vi "CRYRun Project.vi"(2 "Calibrate? (F)":bool, 12 "Do not display panel (F)":bool) -> ()   [LabVIEW 2013]
uses:
  Typedef Control/CRYResult Cluster.ctl
  Typedef Control/CRYTS.ctl
  Typedef Control/CRYStep.ctl
  CRYProject Run Control Global.vi
  Data/CRYData & result stacks global.vi
  CRYMainGlobal.vi
  Calibration/SubVI/CRYCal Global.vi
  CRYProject/CRYProject Editor Global.vi
  Misc/SubVI/CRYMisc vis settings global.vi
  CRYWindow/SubVI/CRYMain Sub Window Global.vi
  Statistics/CRYStatistics Global.vi
panel:
  out "Seq running Ref":refnum<vi>
  out "Seq cont border Ref":refnum<vi>
  out "Seq Continue Ref":refnum<vi>
  out "Verdict Ref":refnum<vi>
  out "Margin Ref":refnum<vi>
  out "Category Name Ref":refnum<vi>
  in  "Updateflg":bool
  in  "VerdictLabel":string
  out "Elapsed Ref":refnum<vi>
  in  "Time Out":bool
  out "Step Name":string
  in  "Verdict":bool caption="°¬ü¬,1Áõ¬,äÂ(Ó"
  out "Step Setup VI No":u32
  out "Margin":dbl format="%#_6p"
  out "Category Name":string
  out "Project Name":string
  in  "done call":bool
  in  "Abort":bool
  in  "Continue":bool
  in  "running":bool
  out "cont border":bool
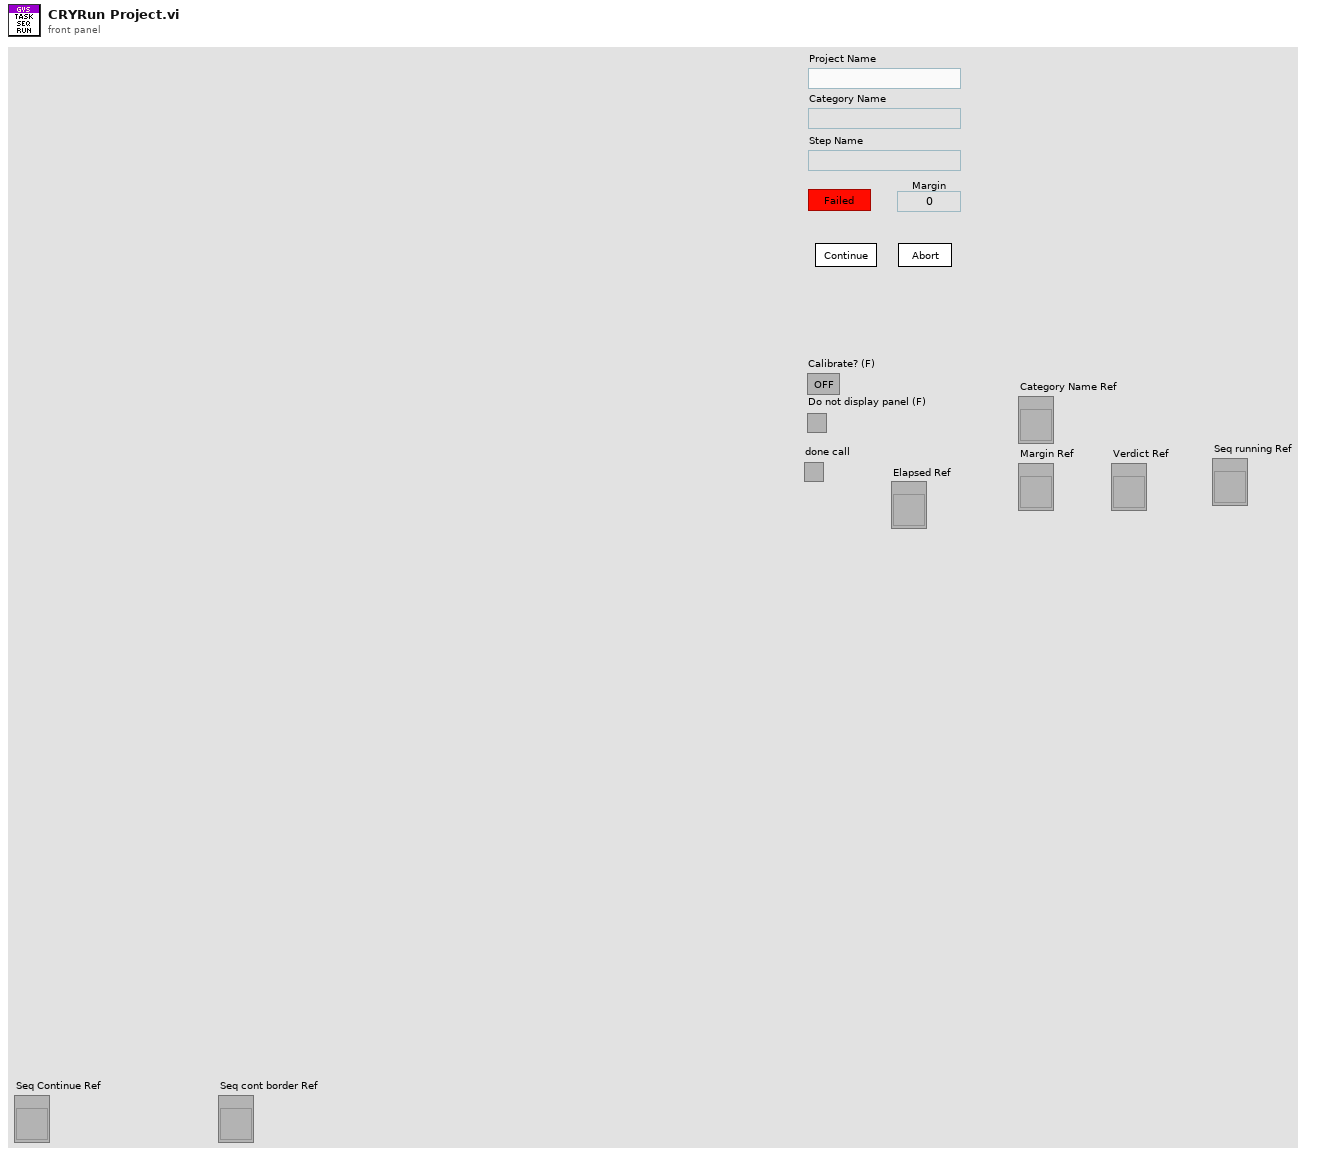
[diagram p1: front panel]
types:
  T1 = typedef "CRYStep.ctl" = cluster{"No.VI":i32, "Category":string, "StepName":string, "Seq setup flattened":string, "Comment":string, "Steps config.":bool[], "Jump config":i32[], "Start":dbl, "Increment":dbl, "Name":string, "Unit":string, "Y data":u16, "Y prefix":string, "Y dB ref":dbl, "Y unit":string, "Repeat State Array":cluster{"Start":dbl, "Increment":dbl, "Count":i32, "Num":i32}[]}
  T2 = typedef "CRYTS.ctl" = cluster{"No.TS":u16, "TS File Path":path, "TS Name":string, "EditStepName":string, "Steps":T1[], "New State":bool, "Change State":bool, "Flattened CurveLib Data":string, "Document Data":string, "EditStepNo":u16, "Operator Start File":string, "Sequence Type":string, "Sequence Language":string}
  T3 = cluster{"Category Name Ref":refnum<vi>, "Step Name Ref":refnum<vi>, "Verdict Ref":refnum<vi>, "Seq Continue Ref":refnum<vi>, "Seq cont border Ref":refnum<vi>, "Seq running Ref":refnum<vi>}
  T4 = typedef "CRYStart Cluster.ctl" = cluster{"SequenceName":string, "Preload Stimulus":bool, "CloseOpenedDisplay":bool, "ClearMeasuredData":bool, "UpdateDisplayDuringRun":bool, "DisplayForConfirmation":bool, "HaltOnFail":bool, "UseSameHardware":bool, "UseSameCalibration":bool}
  T5 = typedef "CRYResult Cluster.ctl" = cluster{"Name":string, "Margin":dbl, "unit":string, "Verdict":bool, "Limit":string, "Max/Min":string, "protected":bool, "Step No.":i32, "Test Info":string, "AutoProtect":bool}
  T6 = typedef "GVSResult Cluster.ctl" = cluster{"Name":string, "Margin":dbl, "unit":string, "Verdict":bool, "Limit":string, "Max/Min":string, "protected":bool, "Step No.":i32, "Test Info":string, "AutoProtect":bool}
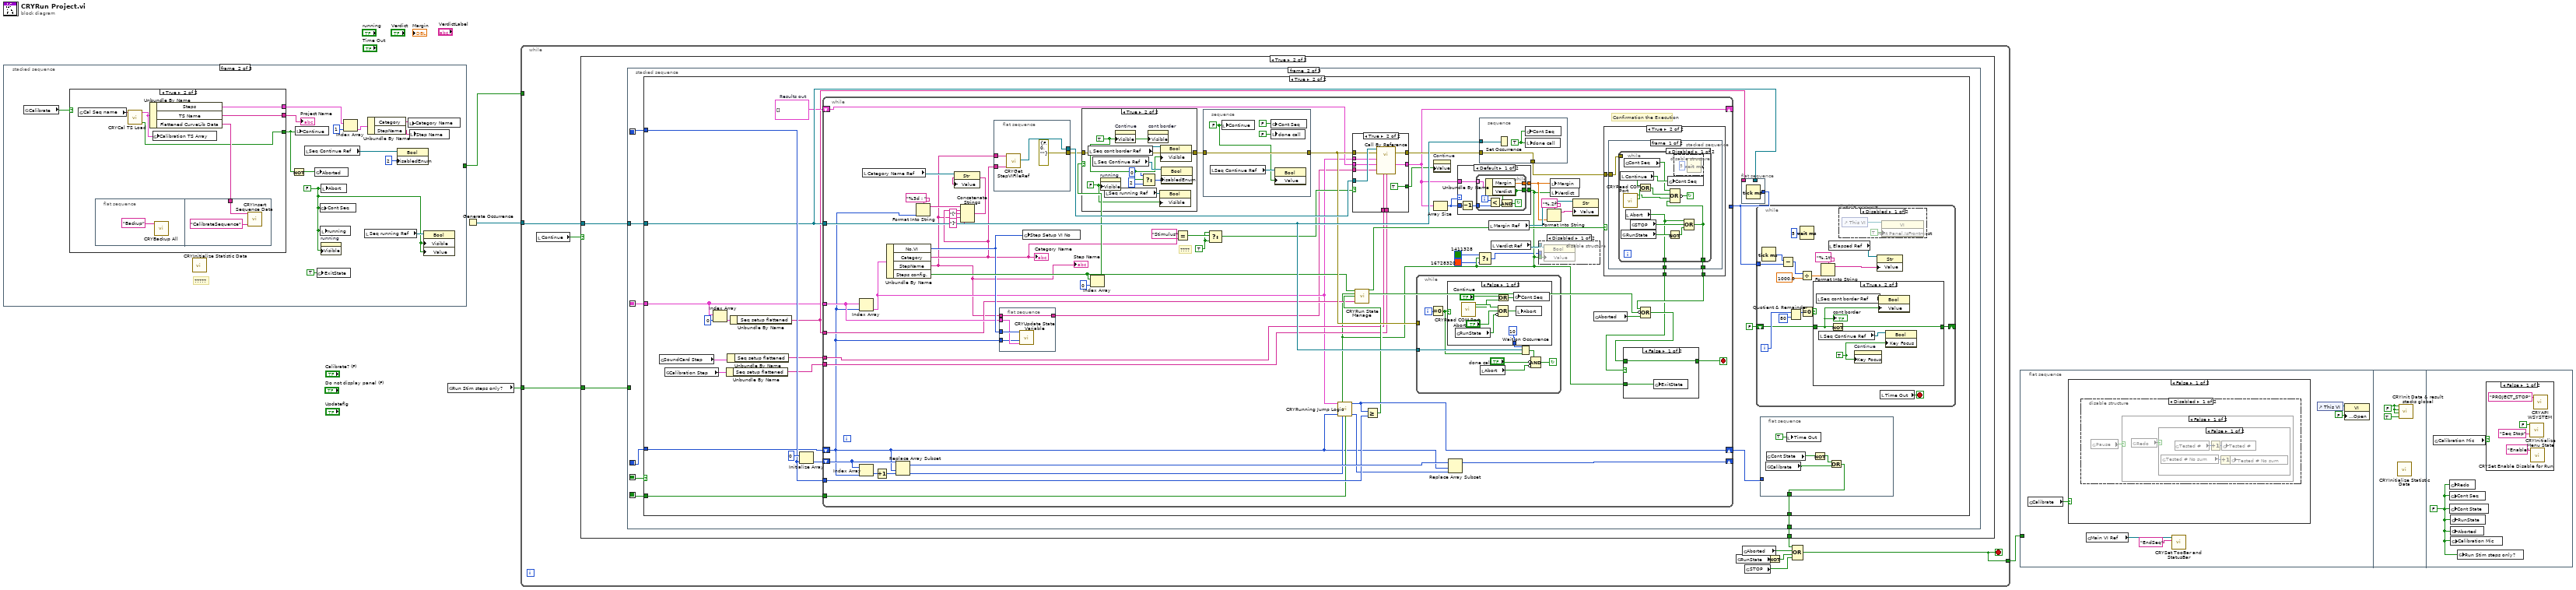
[diagram p0: block diagram]
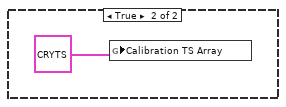
[diagram p5: hidden frame]
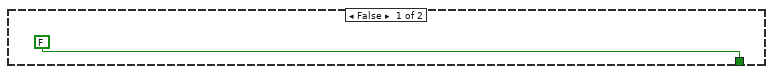
[diagram p7: hidden frame]
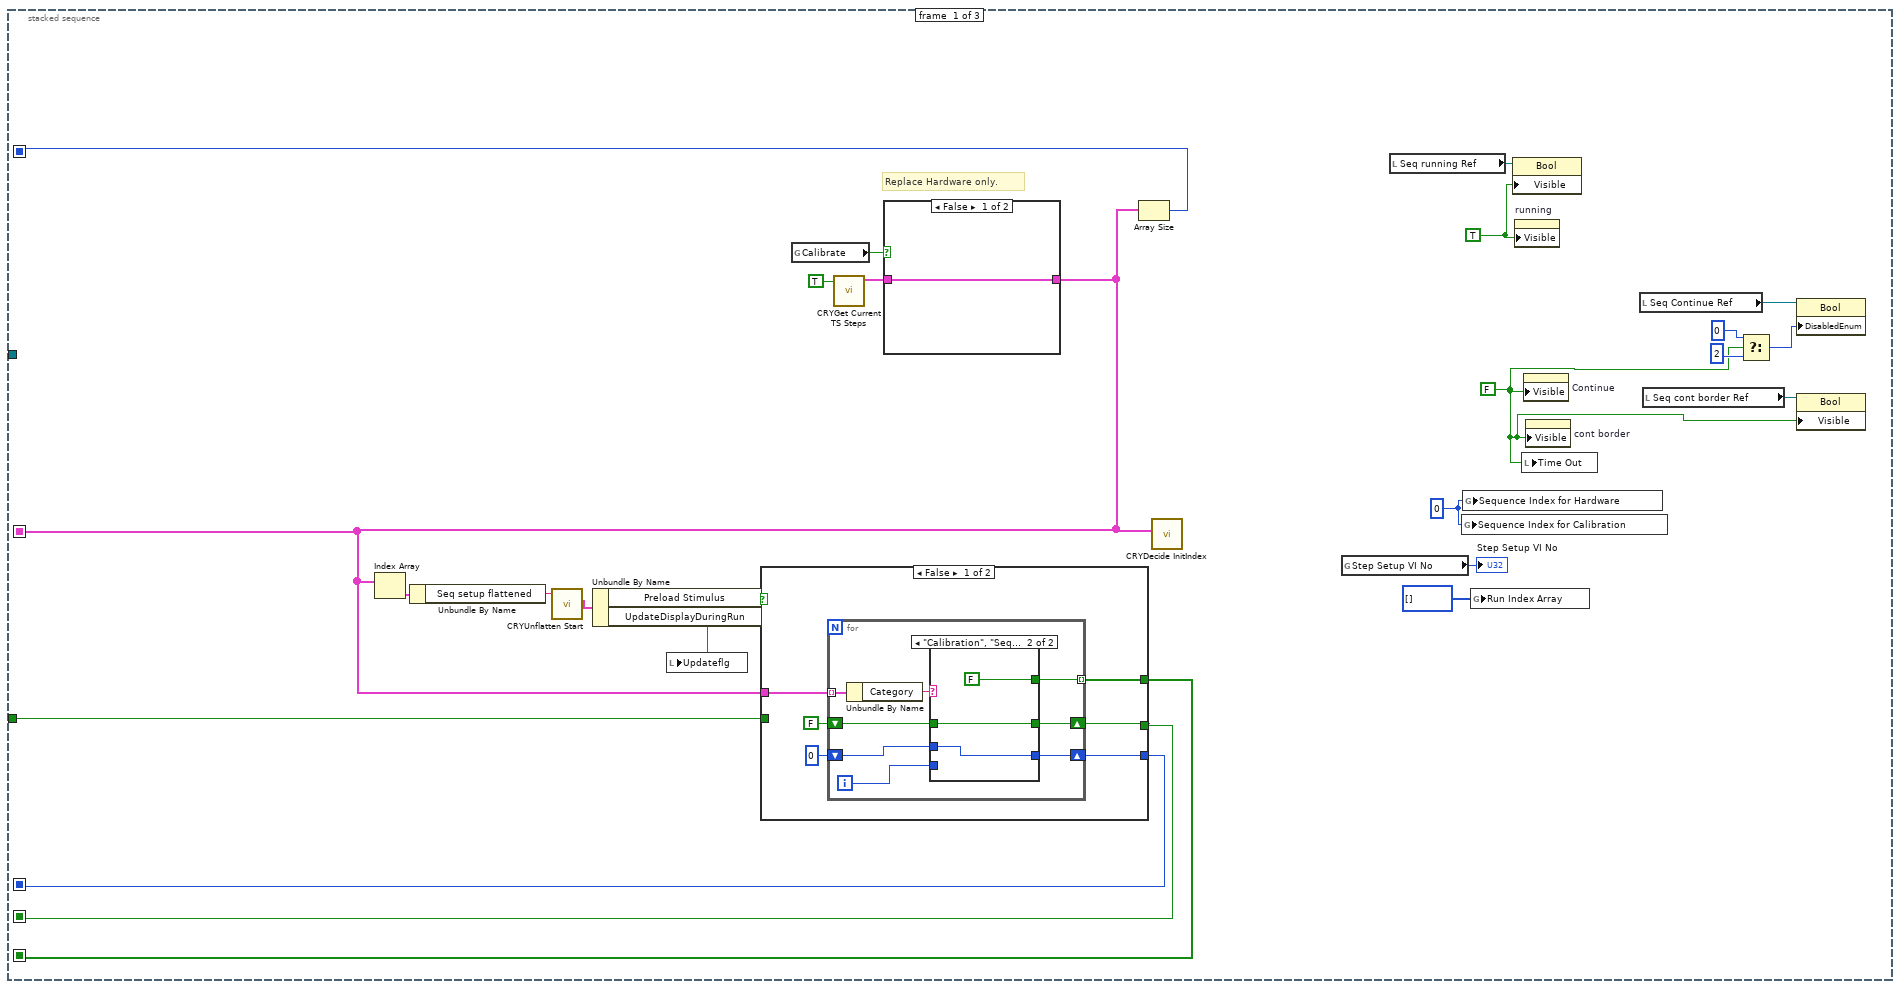
[diagram p8: hidden frame]
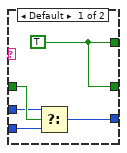
[diagram p9: hidden frame]
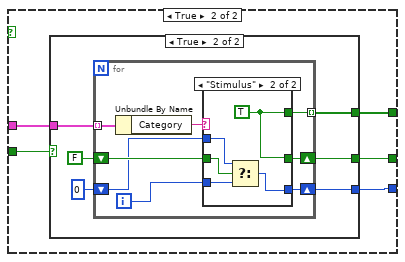
[diagram p10: hidden frame]
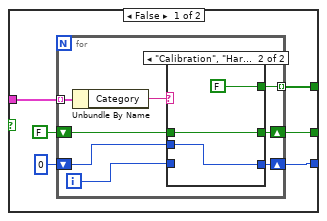
[diagram p11: hidden frame]
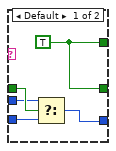
[diagram p12: hidden frame]
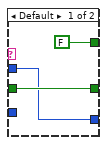
[diagram p13: hidden frame]
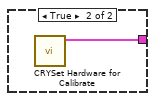
[diagram p14: hidden frame]
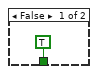
[diagram p15: hidden frame]
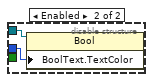
[diagram p18: hidden frame]
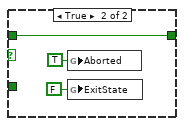
[diagram p19: hidden frame]
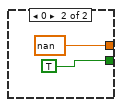
[diagram p20: hidden frame]
diagram:
  n1 = stacked-sequence {
    tunnel: [_ _ w71] -> w3
    frame #0 {
      w11 = TRUE ("Verdict")
      n2 = control-ref of="This VI"() -> (w10:refnum<vi>)
      n3 = call "CRYSet Run Project Front Panel.vi"("Vi Ref in"=w10) -> ()  [unwired: 10 in, 1 out]
      n4 = call "CRYOperator Process.vi"("sAction"="RunCloseAll") -> ()  [unwired: 10 in, 1 out]
      n5 = local write "Verdict"(w11) -> ()
      n6 = global write "CRYProject Run Control Global.vi" "RunState"(w11) -> ()
      n7 = global read "CRYCal Global.vi" "Calibration Mic"() -> (w7:bool)
      n8 = control-ref of="Abort"() -> (w9:refnum<vi>)
      n9 = control-ref of="Continue"() -> (w8:refnum<vi>)
      n10 = global write "CRYData & result stacks global.vi" "Tested # No sum"(u16 0 ("Tested # No sum")) -> ()
      n11 = global write "CRYMainGlobal.vi" "Seq Continue Ref"(w8) -> ()
      n12 = global write "CRYMainGlobal.vi" "Seq Abort Ref"(w9) -> ()
      n13 = case shown="False" w7 {
        frame False {
          n14 = call "CRYInitialize Menu State.vi"("sAction"="Seq Run", "Is Disable?"=TRUE) -> ()  [unwired: 10 in]
          n15 = call "CRYAPI WSYSTEM.vi"("sAction"="PROJECT_RUN") -> ()  [unwired: 7 in, 4 out]
          n16 = call "CRYSet Enable Disable for Run.vi"("sOption"="Disable") -> ()  [unwired: 15 in]
        }
        frame True {
        }
      }
    }
    frame #1 {
      w19 = FALSE
      # "?????"
      n17 = global read "CRYCal Global.vi" "Calibrate"() -> (w29:bool)
      n18 = case shown="True" w29 {
        tunnel: [TRUE ("cont button") w50] -> w17
        tunnel: [w32 w54] -> w27
        tunnel: [w33 w53] -> w28
        frame False {
          n19 = call "CRYGet Current TS Steps.vi"() -> ("TS Name"=w33:string, "Steps"=w32:T1[])  [unwired: 7 in, 3 out]
          n20 = for {
            tunnel: w32 -> [w36] mode=indexing
            shift-right: [w41] -> w30
            shift-left: i32[] [] -> [w40]
            n21 = Unbundle By Name(w36) -> ("Category"=w43:string, "No.VI"=w42:i32, "Steps config."=w39:bool[], "Start"=w35:dbl)
            n22 = Index Array(array=w39, index=6) -> (element=w37:bool)
            n23 = case shown="Default" w43 {
              tunnel: w42 -> [w47 _]
              tunnel: [w46 w49] -> w41
              tunnel: w40 -> [w48 w49]
              frame Default {
                n24 = Build Array (concatenate)(w48, w47) -> (w46:i32[])
              }
              frame "Calibration", "Stimulus" {
              }
            }
            n25 = case shown="True" w37 {
              tunnel: w36 -> [_ w45]
              tunnel: w35 -> [_ w44]
              frame False {
              }
              frame True {
                n26 = call "CRYUpdate Curve from Jump.vi"("Y Value"=w44, "Step Configure"=w45) -> ()  [unwired: 9 in, 1 out]
              }
            }
          }
          n27 = call "CRYDelete Step Data.vi"("Step No"=w30) -> ()  [unwired: 11 in]
        }
        frame True {
          n28 = global read "CRYCal Global.vi" "Cal Seq name"() -> (w55:string)
          n29 = flat-sequence {
            tunnel: w51 -> [w58]
            frame #0 {
              n30 = call "CRYBackup All.vi"("sOption"="Backup") -> ()  [unwired: 11 in]
            }
            frame #1 {
              n31 = call "CRYInsert Sequence Data.vi"("sOption"="CalibrateSequence", "sFlattenedCurveData"=w58) -> ()  [unwired: 8 in, 2 out]
            }
          }
          n32 = call "CRYCal TS Load.vi"("Cal seq name"=w55) -> ("Cal sequence"=w52:T2, "status"=w50:bool)  [unwired: 8 out]
          n33 = Unbundle By Name(w52) -> ("Steps"=w54:T1[], "TS Name"=w53:string, "Flattened CurveLib Data"=w51:string)
          n34 = global write "CRYProject Editor Global.vi" "Calibration TS Array"(w52) -> ()
        }
      }
      "Project Name" <- w28
      n35 = call "CRYInitialize Statistic Data.vi"() -> ()  [unwired: 12 in]
      n36 = Not(x=w17) -> (.not. x?=w16:bool)
      n37 = local write "Continue"(w17) -> ()
      n38 = local read "Seq Continue Ref"() -> (w21:refnum<vi>)
      n39 = global write "CRYProject Run Control Global.vi" "Aborted"(w16) -> ()
      n40 = global write "CRYProject Run Control Global.vi" "ExitState"(TRUE ("ExitState")) -> ()
      n41 = global write "CRYProject Run Control Global.vi" "Cont Seq"(w19) -> ()
      n42 = local write "running"(w19) -> ()
      n43 = property on="running" class="Bool (strict)"("Visible"=w19) -> ()  [unwired: 2 in, 2 out]
      n44 = local write "Abort"(w19) -> ()
      n45 = Index Array(array=w27, index=1) -> (element=w24:T1)
      n46 = local read "Seq running Ref"() -> (w20:refnum<vi>)
      n47 = Unbundle By Name(w24) -> ("Category"=w23:string, "StepName"=w22:string)
      n48 = property class="Bool"(reference=w21, "DisabledEnum"=u8 2) -> ()  [unwired: 1 in, 2 out]
      n49 = local write "Category Name"(w23) -> ()
      n50 = local write "Step Name"(w22) -> ()
      n51 = property class="Bool"(reference=w20, "Visible"=w19, "Value"=w19) -> ()  [unwired: 1 in, 2 out]
    }
    frame #2 {
      n52 = global read "CRYCal Global.vi" "Calibrate"() -> (w71:bool)
      n53 = global write "CRYMisc vis settings global.vi" "Menu?"(FALSE ("Menu?")) -> ()
      n54 = global read "CRYMain Sub Window Global.vi" "Main VI Ref"() -> (w70:refnum<vi>)
      n55 = call "CRYSet TooBar and StatusBar.vi"("Type"="StartSeq", "MainVI Ref In"=w70) -> ("output cluster"=w67:T3, "Elapsed Ref"=→"Elapsed Ref":refnum<vi>)  [unwired: 7 in, 1 out]
      n56 = local read "Verdict"() -> (w64:bool)
      n57 = Unbundle(w67) -> ("Category Name Ref"=→"Category Name Ref":refnum<vi>, "Step Name Ref"=→"Margin Ref":refnum<vi>, "Verdict Ref"=w63:refnum<vi>, "Seq Continue Ref"=→"Seq Continue Ref":refnum<vi>, "Seq cont border Ref"=→"Seq cont border Ref":refnum<vi>, "Seq running Ref"=→"Seq running Ref":refnum<vi>)
      "Verdict Ref" <- w63
      n58 = property class="Bool"(reference=w63, "Value"=w64) -> ()  [unwired: 1 in, 2 out]
      n59 = property on="Verdict" class="Bool (strict)"() -> ("Strings [4]"=w62:string[])  [unwired: 2 in, 2 out]
      n60 = property class="Bool"(reference=w63, "Strings [4]"=w62) -> ()  [unwired: 1 in, 2 out]
    }
  }
  n61 = global read "CRYProject Run Control Global.vi" "Run Stim steps only?"() -> (w2:bool)
  n62 = Generate Occurrence() -> (w4:refnum<k4>)
  n63 = while {
    tunnel: w4 -> [w81]
    tunnel: w3 -> [_]
    tunnel: w2 -> [w74]
    tunnel: [w73] -> w1
    stop <- w73 stop-if-true
    n64 = local read "Continue"() -> (w80:bool)
    n65 = case shown="True" w80 {
      tunnel: w81 -> [_ w85]
      tunnel: [FALSE ("abort button") w84] -> w76
      tunnel: w74 -> [_ w83]
      frame False {
      }
      frame True {
        n66 = stacked-sequence {
          seq-local: [w106 _ _] -> [_ w187 _]
          seq-local: [w86 _ _] -> [_ w189 _]
          seq-local: [w100 _ _] -> [_ w186 _]
          seq-local: [w98 _ _] -> [_ w185 _]
          seq-local: [w96 _ _] -> [_ w184 _]
          tunnel: w85 -> [_ w190 _]
          tunnel: [_ w188 _] -> w84
          tunnel: w83 -> [w99 _ _]
          frame #0 {
            w105 = 0 ("Sequence Index for Hardware")
            w88 = FALSE ("Visible")
            w91 = TRUE ("Visible")
            # "Replace Hardware only."
            n67 = global read "CRYCal Global.vi" "Calibrate"() -> (w109:bool)
            n68 = call "CRYGet Current TS Steps.vi"("Current Only?"=TRUE) -> ("Steps"=w108:T1[])  [unwired: 6 in, 4 out]
            n69 = case shown="False" w109 {
              tunnel: [w182 w183] -> w86
              tunnel: w108 -> [w182 _]
              frame False {
              }
              frame True {
                n70 = call "CRYSet Hardware for Calibrate.vi"() -> ("Steps Out"=w183:T1[])  [unwired: 11 in]
              }
            }
            n71 = Index Array(array=w86) -> (element=w104:T1)  [unwired: 1 in]
            n72 = Unbundle By Name(w104) -> ("Seq setup flattened"=w103:string)
            n73 = call "CRYUnflatten Start.vi"("Unflatten Sequence"=w103) -> ("Sequence Configure"=w102:T4)  [unwired: 8 in, 2 out]
            n74 = Unbundle By Name(w102) -> ("Preload Stimulus"=w101:bool, "UpdateDisplayDuringRun"=w97:bool)
            n75 = local write "Updateflg"(w97) -> ()
            n76 = case shown="False" w101 {
              tunnel: w86 -> [w116 w136]
              tunnel: [w115 w135] -> w100
              tunnel: w99 -> [_ w137]
              tunnel: [w113 w134] -> w98
              tunnel: [w111 w133] -> w96
              frame False {
                n77 = for {
                  tunnel: w116 -> [w124] mode=indexing
                  tunnel: [w122] -> w115 mode=indexing
                  shift-right: [w120] -> w113
                  shift-left: FALSE -> [w121]
                  shift-right: [w118] -> w111
                  shift-left: 0 -> [w117]
                  i -> [w119]
                  n78 = Unbundle By Name(w124) -> ("Category"=w123:string)
                  n79 = case shown="\"Calibration\", \"Sequence\", \"SoundCard\"" w123 {
                    tunnel: [w129 FALSE] -> w122
                    tunnel: w121 -> [w128 w131]
                    tunnel: [w129 w131] -> w120
                    tunnel: w119 -> [w127 _]
                    tunnel: [w126 w130] -> w118
                    tunnel: w117 -> [w125 w130]
                    frame Default {
                      w129 = TRUE
                      n80 = Select(t=w125, s=w128, f=w127) -> (s? t:f=w126:i32)
                    }
                    frame "Calibration", "Sequence", "SoundCard" {
                    }
                  }
                }
              }
              frame True {
                n81 = case shown="True" w137 {
                  tunnel: w136 -> [w143 w165]
                  tunnel: [w142 w164] -> w135
                  tunnel: [w140 w162] -> w134
                  tunnel: [w138 w160] -> w133
                  frame False {
                    n82 = for {
                      tunnel: w143 -> [w151] mode=indexing
                      tunnel: [w149] -> w142 mode=indexing
                      shift-right: [w147] -> w140
                      shift-left: FALSE -> [w148]
                      shift-right: [w144] -> w138
                      shift-left: 0 -> [w145]
                      i -> [w146]
                      n83 = Unbundle By Name(w151) -> ("Category"=w150:string)
                      n84 = case shown="\"Calibration\", \"Hardware\", \"Sequence\", \"Stimulus\"" w150 {
                        tunnel: [w156 FALSE] -> w149
                        tunnel: w148 -> [w155 w158]
                        tunnel: [w156 w158] -> w147
                        tunnel: w146 -> [w154 _]
                        tunnel: w145 -> [w153 w157]
                        tunnel: [w152 w157] -> w144
                        frame Default {
                          w156 = TRUE
                          n85 = Select(t=w153, s=w155, f=w154) -> (s? t:f=w152:i32)
                        }
                        frame "Calibration", "Hardware", "Sequence", "Stimulus" {
                        }
                      }
                    }
                  }
                  frame True {
                    n86 = for {
                      tunnel: w165 -> [w173] mode=indexing
                      tunnel: [w171] -> w164 mode=indexing
                      shift-right: [w169] -> w162
                      shift-left: FALSE -> [w170]
                      shift-right: [w166] -> w160
                      shift-left: 0 -> [w167]
                      i -> [w168]
                      n87 = Unbundle By Name(w173) -> ("Category"=w172:string)
                      n88 = case shown="\"Stimulus\"" w172 {
                        tunnel: [FALSE w181] -> w171
                        tunnel: w170 -> [w175 w180]
                        tunnel: [w175 w181] -> w169
                        tunnel: w168 -> [_ w179]
                        tunnel: w167 -> [w174 w178]
                        tunnel: [w174 w177] -> w166
                        frame Default {
                        }
                        frame "Stimulus" {
                          w181 = TRUE
                          n89 = Select(t=w178, s=w180, f=w179) -> (s? t:f=w177:i32)
                        }
                      }
                    }
                  }
                }
              }
            }
            n90 = Array Size(array=w86) -> (size(s)=w106:i32)
            n91 = call "CRYDecide InitIndex.vi"("Steps In"=w86) -> ()  [unwired: 11 in]
            n92 = global read "CRYProject Editor Global.vi" "Step Setup VI No"() -> (→"Step Setup VI No":i32)
            n93 = local read "Seq running Ref"() -> (w92:refnum<vi>)
            n94 = global write "CRYProject Editor Global.vi" "Sequence Index for Calibration"(w105) -> ()
            n95 = global write "CRYProject Editor Global.vi" "Sequence Index for Hardware"(w105) -> ()
            n96 = global write "CRYProject Run Control Global.vi" "Run Index Array"(u32[] [] ("Run Index Array")) -> ()
            n97 = property class="Bool"(reference=w92, "Visible"=w91) -> ()  [unwired: 1 in, 2 out]
            n98 = property on="running" class="Bool (strict)"("Visible"=w91) -> ()  [unwired: 2 in, 2 out]
            n99 = local write "Time Out"(w88) -> ()
            n100 = property on="Continue" class="Bool (strict)"("Visible"=w88) -> ()  [unwired: 2 in, 2 out]
            n101 = property on="cont border" class="Bool (strict)"("Visible"=w88) -> ()  [unwired: 2 in, 2 out]
            n102 = local read "Seq Continue Ref"() -> (w94:refnum<vi>)
            n103 = local read "Seq cont border Ref"() -> (w93:refnum<vi>)
            n104 = Select(t=u8 0, s=w88, f=u8 2) -> (s? t:f=w87:u8)
            n105 = property class="Bool"(reference=w94, "DisabledEnum"=w87) -> ()  [unwired: 1 in, 2 out]
            n106 = property class="Bool"(reference=w93, "Visible"=w88) -> ()  [unwired: 1 in, 2 out]
          }
          frame #1 {
            n107 = case shown="True" w185 {
              tunnel: w190 -> [_ w203]
              tunnel: w189 -> [_ w198]
              tunnel: [TRUE w210] -> w188
              tunnel: w187 -> [_ w207]
              tunnel: w186 -> [_ w206]
              tunnel: w184 -> [_ w205]
              frame False {
              }
              frame True {
                w200 = T5[] []  # Results out
                n108 = global read "CRYProject Editor Global.vi" "SoundCard Step"() -> (w194:T1)
                n109 = global read "CRYProject Editor Global.vi" "Calibration Step"() -> (w195:T1)
                n110 = Index Array(array=w198, index=0) -> (element=w201:T1)
                n111 = Unbundle By Name(w195) -> ("Seq setup flattened"=w192:string)
                n112 = Unbundle By Name(w194) -> ("Seq setup flattened"=w193:string)
                n113 = Unbundle By Name(w201) -> ("Seq setup flattened"=w199:string)
                n114 = Initialize Array(0 ("step execution\ncounter"), w207) -> (w208:i32[])
                n115 = while {
                  tunnel: w203 -> [w295]
                  tunnel: w198 -> [w273]
                  shift-right: [w283] -> w204
                  shift-left: w205 -> [w237]
                  tunnel: w207 -> [w282]
                  shift-right: [w271] -> _
                  shift-left: w208 -> [w286]
                  tunnel: w206 -> [w281]
                  tunnel: w199 -> [w261]
                  shift-right: [w260] -> _
                  shift-left: w200 -> [w259]
                  tunnel: w193 -> [w258]
                  tunnel: w192 -> [w257]
                  tunnel: w197 -> [_]
                  stop <- w267 stop-if-true
                  w262 = TRUE
                  # "????"
                  # "Confirmation the Execution"
                  n116 = Index Array(array=w273, index=w237) -> (element=w256:T1)
                  n117 = Index Array(array=w286, index=w237) -> (element=w287:i32)
                  n118 = local read "Category Name Ref"() -> (w254:refnum<vi>)
                  n119 = Increment(x=w287) -> (x+1=w284:i32)
                  n120 = Unbundle By Name(w256) -> ("No.VI"=w274:i32, "Category"=w251:string, "StepName"=w236:string, "Steps config."=w279:bool[])
                  "Category Name" <- w251
                  "Step Name" <- w236
                  n121 = Replace Array Subset(array=w286, new element=w284, index=w237) -> (w285:i32[])
                  n122 = Format Into String(format string="%3d : ", w237) -> (resulting string=w240:string)  [unwired: 2 in, 1 out]
                  n123 = Concatenate Strings(w240, w251, "[" ("string"), w236, "]" ("string")) -> (w248:string)
                  n124 = property class="Str"(reference=w254, "Value"=w248) -> ()  [unwired: 1 in, 2 out]
                  n125 = flat-sequence {
                    tunnel: [w312] -> w294
                    tunnel: [errorcluster {"status"=FALSE, "code"=0, "source"=""} ("error out")] -> w291
                    tunnel: w251 -> [w310]
                    tunnel: w236 -> [w309]
                    frame #0 {
                      n126 = call "CRYGet StepVIFileRef.vi"("Category"=w310, "Step Name"=w309) -> ("Step Run VI ref"=w312:refnum<vi>)  [unwired: 6 in, 2 out]
                    }
                  }
                  n127 = flat-sequence {
                    tunnel: w274 -> [w308]
                    tunnel: w273 -> [w307]
                    tunnel: w237 -> [w306]
                    tunnel: w236 -> [w305]
                    tunnel: [w305] -> w255
                    frame #0 {
                      n128 = call "CRYUpdate State Variable.vi"("Step VI No In"=w308, "Step Index"=w306, "Steps"=w307) -> ()  [unwired: 12 in, 1 out]
                    }
                  }
                  n129 = global write "CRYProject Editor Global.vi" "Step Setup VI No"(w274) -> ()
                  n130 = Index Array(array=w279, index=0) -> (element=w278:bool)
                  n131 = case shown="True" w278 {
                    tunnel: [w339 w348] -> w290
                    tunnel: w291 -> [w339 w348]
                    frame False {
                    }
                    frame True {
                      w343 = TRUE ("Visible")
                      w344 = FALSE ("Visible")
                      n132 = local read "Seq cont border Ref"() -> (w346:refnum<vi>)
                      n133 = local read "Seq Continue Ref"() -> (w347:refnum<vi>)
                      n134 = property on="running" class="Bool (strict)"("Visible"=w344) -> ()  [unwired: 2 in, 2 out]
                      n135 = local read "Seq running Ref"() -> (w345:refnum<vi>)
                      n136 = property on="Continue" class="Bool (strict)"("Visible"=w343) -> ()  [unwired: 2 in, 2 out]
                      n137 = Select(t=u8 0, s=w343, f=u8 2) -> (s? t:f=w340:u8)
                      n138 = property on="cont border" class="Bool (strict)"("Visible"=w343) -> ()  [unwired: 2 in, 2 out]
                      n139 = property class="Bool"(reference=w345, "Visible"=w344) -> ()  [unwired: 1 in, 2 out]
                      n140 = property class="Bool"(reference=w346, "Visible"=w343) -> ()  [unwired: 1 in, 2 out]
                      n141 = property class="Bool"(reference=w347, "DisabledEnum"=w340) -> ()  [unwired: 1 in, 2 out]
                    }
                  }
                  n142 = Equal?(x="Stimulus", y=w251) -> (x = y?=w264:bool)
                  n143 = stacked-sequence {
                    tunnel: w290 -> [w405]
                    tunnel: [w405] -> w293
                    frame #0 {
                      w401 = FALSE ("cont button")
                      n144 = local read "Seq Continue Ref"() -> (w402:refnum<vi>)
                      n145 = local write "Continue"(w401) -> ()
                      n146 = global write "CRYProject Run Control Global.vi" "Cont Seq"(FALSE ("Cont Seq")) -> ()
                      n147 = local write "done call"(FALSE ("done call")) -> ()
                      n148 = property class="Bool"(reference=w402, "Value"=w401) -> ()  [unwired: 1 in, 2 out]
                    }
                  }
                  n149 = Select(t=w262, s=w264, f=w262) -> (s? t:f=w263:bool)
                  n150 = case shown="True" w263 {
                    tunnel: w294 -> [_ w338]
                    tunnel: w293 -> [w328 w337]
                    tunnel: w258 -> [_ w333]
                    tunnel: w257 -> [_ w334]
                    tunnel: w256 -> [_ w332]
                    tunnel: w255 -> [_ w330]
                    tunnel: [w328 w336] -> w292
                    tunnel: [_ w335] -> w260
                    tunnel: w259 -> [_ w331]
                    tunnel: [FALSE ("Continue") TRUE ("Continue")] -> w238
                    frame False {
                    }
                    frame True {
                      n151 = call-by-ref "?"(reference=w338, error in=w337, "Setup in"=w332, "Results in"=w331, "Step name"=w330, "Hardware in"=w333, "Calibration in"=w334) -> (error out=w336:errorcluster, "Results out"=w335:T6[])  [unwired: 6 in, 5 out]
                    }
                  }
                  n152 = while {
                    tunnel: w295 -> [w387]
                    tunnel: w293 -> [_]
                    i -> [w388]
                    stop <- w382 continue-if-true
                    n153 = Equal To 0?(x=w388) -> (x = 0?=w385:bool)
                    n154 = case shown="False" w385 {
                      tunnel: [10 ("ms timeout (-1)") 2 ("ms timeout (-1)")] -> w386
                      frame False {
                        n155 = global read "CRYProject Run Control Global.vi" "RunState"() -> (w390:bool)
                        n156 = call "CRYRead COM Port.vi"() -> ("State 2 (Start & Continue)"=w394:bool, "State (Redo & Abort)"=w396:bool)  [unwired: 5 in, 5 out]
                        n157 = Or(x="Continue", y=w394) -> (x .or. y?=w392:bool)
                        n158 = Compound Arithmetic op=OR(w396, "Abort", invert w390) -> (w389:bool)
                        n159 = global write "CRYProject Run Control Global.vi" "Cont Seq"(w392) -> ()
                        n160 = local write "Abort"(w389) -> ()
                      }
                      frame True {
                      }
                    }
                    n161 = local read "Abort"() -> (w381:bool)
                    n162 = Wait on Occurrence(1:w385, 2:w387, 3:w386) -> (0:w383:bool)
                    n163 = Compound Arithmetic op=AND(w383, invert "done call", invert w381) -> (w382:bool)
                  }
                  n164 = property on="Continue" class="Bool (strict)"("Value"=w238) -> ()  [unwired: 2 in, 2 out]
                  n165 = Array Size(array=w260) -> (size(s)=w280:i32)
                  n166 = case shown="Default" w280 {
                    tunnel: [w317 nan ("Margin")] -> w246
                    tunnel: w280 -> [w316 _]
                    tunnel: [w314 TRUE ("Verdict")] -> w244
                    tunnel: w260 -> [w313 _]
                    frame Default {
                      n167 = Decrement(x=w316) -> (x-1=w315:i32)
                      n168 = while {
                        tunnel: w315 -> [w323]
                        tunnel: [w320] -> w314
                        tunnel: [w324] -> w317
                        tunnel: w313 -> [w318] mode=indexing
                        i -> [w322]
                        stop <- w319 continue-if-true
                        n169 = Unbundle By Name(w318) -> ("Margin"=w324:dbl, "Verdict"=w320:bool)
                        n170 = Less?(x=w322, y=w323) -> (x < y?=w321:bool)
                        n171 = And(x=w320, y=w321) -> (x .and. y?=w319:bool)
                      }
                    }
                    frame 0 {
                    }
                  }
                  n172 = call "CRYRunning Jump Logic.vi"("Step Configure"=w256, "Pass?"=w244, "Step pointer in"=w237, "Step execution count"=w284, "Allowed-to-run steps mask"=w281) -> ("Step pointer out"=w283:i32, "execution count out"=w270:i32)  [unwired: 9 in]
                  n173 = Greater Or Equal?(x=w283, y=w282) -> (x >= y?=w277:bool)
                  n174 = call "CRYRun State Manage.vi"("Steps config."=w279, "Pass?"=w244, "Last step?"=w277, "Seq setup flattened"=w261) -> ("Wait for confirmation"=w275:bool, "Continue Sequence"=w276:bool)  [unwired: 10 in]
                  n175 = Replace Array Subset(array=w285, new element=w270, index=w237) -> (w271:i32[])
                  n176 = Select(t=u32 1411328 ("Boolean Text.Text Colors:Text Color"), s=w244, f=u32 16728320 ("Boolean Text.Text Colors:Text Color")) -> (s? t:f=w241:u32)
                  n177 = stacked-sequence {
                    tunnel: w292 -> [w399]
                    tunnel: w295 -> [w400]
                    tunnel: [w399] -> w288
                    frame #0 {
                      w398 = TRUE ("done call")
                      n178 = Set Occurrence(w400) -> ()
                      n179 = global write "CRYProject Run Control Global.vi" "Cont Seq"(w398) -> ()
                      n180 = local write "done call"(w398) -> ()
                    }
                  }
                  n181 = local read "Margin Ref"() -> (w252:refnum<vi>)
                  n182 = local read "Verdict Ref"() -> (w253:refnum<vi>)
                  n183 = disable-structure shown="Disabled" {
                    disable-tunnel: w253 -> [w297 w298]
                    disable-tunnel: w244 -> [w296 _]
                    disable-tunnel: w241 -> [_ w299]
                    frame Disabled {
                      n184 = property class="Bool"(reference=w297, "Value"=w296) -> ()  [unwired: 1 in, 2 out]
                    }
                    frame Enabled {
                      n185 = property class="Bool"(reference=w298, "BoolText.TextColor"=w299) -> ()  [unwired: 1 in, 2 out]
                    }
                  }
                  n186 = Format Into String(format string="%.2f", w246) -> (resulting string=w245:string)  [unwired: 2 in, 1 out]
                  n187 = local write "Margin"(w246) -> ()
                  n188 = local write "Verdict"(w244) -> ()
                  n189 = property class="Str"(reference=w252, "Value"=w245) -> ()  [unwired: 1 in, 2 out]
                  n190 = global read "CRYProject Run Control Global.vi" "Aborted"() -> (w269:bool)
                  n191 = case shown="True" w275 {
                    tunnel: w288 -> [_ w356]
                    tunnel: [w350 w355] -> w289
                    tunnel: [w349 w354] -> w266
                    frame False {
                      n192 = global read "CRYProject Run Control Global.vi" "RunState"() -> (w352:bool)
                      n193 = local read "Abort"() -> (w349:bool)
                      n194 = global read "CRYMainGlobal.vi" "STOP"() -> (w353:bool)
                      n195 = Not(x=w352) -> (.not. x?=w351:bool)
                      n196 = Compound Arithmetic op=OR(w349, w353, w351) -> (w350:bool)
                    }
                    frame True {
                      n197 = stacked-sequence {
                        tunnel: w356 -> [w359 _]
                        tunnel: [w358 _] -> w355
                        tunnel: [w357 _] -> w354
                        frame #0 {
                          n198 = while {
                            tunnel: w359 -> [_]
                            tunnel: [w363] -> w358
                            tunnel: [w360] -> w357
                            stop <- w368 continue-if-true
                            n199 = local read "Continue"() -> (w362:bool)
                            n200 = global read "CRYProject Run Control Global.vi" "RunState"() -> (w365:bool)
                            n201 = call "CRYRead COM Port.vi"() -> ("State 2 (Start & Continue)"=w370:bool, "State (Redo & Abort)"=w367:bool)  [unwired: 5 in, 5 out]
                            n202 = global read "CRYProject Run Control Global.vi" "Cont Seq"() -> (w361:bool)
                            n203 = local read "Abort"() -> (w360:bool)
                            n204 = global read "CRYMainGlobal.vi" "STOP"() -> (w366:bool)
                            n205 = Or(x=w362, y=w370) -> (x .or. y?=w369:bool)
                            n206 = global write "CRYProject Run Control Global.vi" "Cont Seq"(w362) -> ()
                            n207 = Not(x=w365) -> (.not. x?=w364:bool)
                            n208 = disable-structure shown="Disabled" {
                              frame Disabled {
                                n209 = Wait (ms)(milliseconds to wait=u32 5) -> ()  [unwired: 1 out]
                              }
                              frame Enabled {
                              }
                            }
                            n210 = Compound Arithmetic op=OR(w360, w366, w364) -> (w363:bool)
                            n211 = Compound Arithmetic op=OR(w361, w369, w367, w363) -> (invert w368:bool)
                          }
                        }
                        frame #1 {
                          w373 = FALSE ("Visible")
                          w376 = TRUE ("Visible")
                          w378 = FALSE ("cont button")
                          n212 = local read "Seq cont border Ref"() -> (w380:refnum<vi>)
                          n213 = local read "Seq Continue Ref"() -> (w379:refnum<vi>)
                          n214 = local read "Seq running Ref"() -> (w377:refnum<vi>)
                          n215 = property on="running" class="Bool (strict)"("Visible"=w376) -> ()  [unwired: 2 in, 2 out]
                          n216 = property on="Continue" class="Bool (strict)"("Visible"=w373) -> ()  [unwired: 2 in, 2 out]
                          n217 = property on="cont border" class="Bool (strict)"("Visible"=w373) -> ()  [unwired: 2 in, 2 out]
                          n218 = Select(t=u8 0, s=w373, f=u8 2) -> (s? t:f=w372:u8)
                          n219 = property class="Bool"(reference=w377, "Visible"=w376) -> ()  [unwired: 1 in, 2 out]
                          n220 = local write "Continue"(w378) -> ()
                          n221 = property class="Bool"(reference=w379, "DisabledEnum"=w372, "Value"=w378) -> ()  [unwired: 1 in, 2 out]
                          n222 = property class="Bool"(reference=w380, "Visible"=w373) -> ()  [unwired: 1 in, 2 out]
                        }
                      }
                    }
                  }
                  n223 = Compound Arithmetic op=OR(w289, invert w276, w269) -> (w268:bool)
                  n224 = case shown="False" w266 {
                    tunnel: w268 -> [w301 w303]
                    tunnel: [w301 w303] -> w267
                    tunnel: w244 -> [w300 _]
                    frame False {
                      n225 = global write "CRYProject Run Control Global.vi" "ExitState"(w300) -> ()
                    }
                    frame True {
                      n226 = global write "CRYProject Run Control Global.vi" "Aborted"(TRUE ("Aborted")) -> ()
                      n227 = global write "CRYProject Run Control Global.vi" "ExitState"(FALSE ("ExitState")) -> ()
                    }
                  }
                }
                n228 = flat-sequence {
                  tunnel: [w235] -> w197
                  tunnel: w203 -> [_]
                  tunnel: w199 -> [_]
                  frame #0 {
                    n229 = Tick Count (ms)() -> (millisecond timer value=w235:u32)
                  }
                }
                n230 = while {
                  tunnel: w197 -> [w225]
                  shift-right: [w211] -> _
                  shift-left: FALSE -> [w212]
                  i -> [w213]
                  stop <- w224 stop-if-true
                  n231 = Tick Count (ms)() -> (millisecond timer value=w226:u32)
                  n232 = Subtract(x=w226, y=w225) -> (x-y=w219:u32)
                  n233 = Quotient & Remainder(x=w213, y=80) -> (x-y*floor(x/y)=w214:i32)  [unwired: 1 out]
                  n234 = Wait (ms)(milliseconds to wait=u32 5 ("millisecond multiple")) -> ()  [unwired: 1 out]
                  n235 = Divide(x=w219, y=1000.0) -> (x/y=w221:dbl)
                  n236 = Equal To 0?(x=w214) -> (x = 0?=w215:bool)
                  n237 = case shown="True" w215 {
                    tunnel: w212 -> [w229 w232]
                    tunnel: [w229 w234] -> w211
                    frame False {
                    }
                    frame True {
                      w230 = TRUE ("Key Focus")
                      n238 = local read "Seq cont border Ref"() -> (w233:refnum<vi>)
                      n239 = local read "Seq Continue Ref"() -> (w231:refnum<vi>)
                      n240 = Not(x=w232) -> (.not. x?=w234:bool)
                      n241 = property on="Continue" class="Bool (strict)"("Key Focus"=w230) -> ()  [unwired: 2 in, 2 out]
                      n242 = property class="Bool"(reference=w233, "Value"=w232) -> ()  [unwired: 1 in, 2 out]
                      n243 = property class="Bool"(reference=w231, "Key Focus"=w230) -> ()  [unwired: 1 in, 2 out]
                      "cont border" <- w232
                    }
                  }
                  n244 = Format Into String(format string="%.1t", w221) -> (resulting string=w218:string)  [unwired: 2 in, 1 out]
                  n245 = local read "Elapsed Ref"() -> (w217:refnum<vi>)
                  n246 = disable-structure shown="Disabled" {
                    frame Disabled {
                      n247 = control-ref of="This VI"() -> (w228:refnum<vi>)
                      n248 = property class="VI"(reference=w228, "Front Panel.IsFrontmost"=TRUE ("Front Panel Window:Is Frontmost")) -> ()  [unwired: 1 in, 2 out]
                    }
                    frame Enabled {
                    }
                  }
                  n249 = property class="Str"(reference=w217, "Value"=w218) -> ()  [unwired: 1 in, 2 out]
                  n250 = local read "Time Out"() -> (w224:bool)
                }
                n251 = flat-sequence {
                  tunnel: [w410] -> w210
                  tunnel: w204 -> [_]
                  frame #0 {
                    n252 = global read "CRYCal Global.vi" "Calibrate"() -> (w409:bool)
                    n253 = global read "CRYProject Run Control Global.vi" "Cont State"() -> (w407:bool)
                    n254 = local write "Time Out"(TRUE ("Time Out")) -> ()
                    n255 = Not(x=w407) -> (.not. x?=w408:bool)
                    n256 = Or(x=w408, y=w409) -> (x .or. y?=w410:bool)
                  }
                }
              }
            }
          }
          frame #2 {
            n257 = flat-sequence {
              frame #0 {
                n258 = global read "CRYCal Global.vi" "Calibrate"() -> (w411:bool)
                n259 = case shown="False" w411 {
                  frame False {
                    n260 = global read "CRYData & result stacks global.vi" "Pause"() -> (w412:bool)
                    n261 = case shown="False" w412 {
                      frame False {
                        n262 = global read "CRYData & result stacks global.vi" "Redo"() -> (w413:bool)
                        n263 = case shown="False" w413 {
                          frame False {
                            n264 = flat-sequence {
                              tunnel: [w417] -> w414
                              tunnel: w414 -> [w420]
                              frame #0 {
                                n265 = global read "CRYData & result stacks global.vi" "Tested #"() -> (w418:u16)
                                n266 = global read "CRYData & result stacks global.vi" "Tested # No sum"() -> (w415:u16)
                                n267 = Increment(x=w418) -> (x+1=w417:u16)
                                n268 = global write "CRYData & result stacks global.vi" "Tested #"(w417) -> ()
                                n269 = Increment(x=w415) -> (x+1=w416:u16)
                                n270 = global write "CRYData & result stacks global.vi" "Tested # No sum"(w416) -> ()
                              }
                              frame #1 {
                                n271 = global read "CRYMain Sub Window Global.vi" "Main VI Ref"() -> (w419:refnum<vi>)
                                n272 = call "CRYGet String Reference.vi"("Label Name"="Tested:", "VI Refnum"=w419) -> ("String Ref Out"=w422:refnum<vi>)  [unwired: 7 in, 2 out]
                                n273 = Number To Decimal String(number=w420) -> (decimal integer string=w421:string)  [unwired: 1 in]
                                n274 = property class="Str"(reference=w422, "Value"=w421) -> ()  [unwired: 1 in, 2 out]
                              }
                            }
                          }
                          frame True {
                          }
                        }
                      }
                      frame True {
                      }
                    }
                  }
                  frame True {
                  }
                }
              }
              frame #1 {
                w425 = 0 ("Sequence Index for Hardware")
                n275 = local read "Step Setup VI No"() -> (w427:u32)
                n276 = global read "CRYProject Run Control Global.vi" "Cont State"() -> (w426:bool)
                n277 = global write "CRYProject Run Control Global.vi" "Run Index Array"(u32[] [] ("Run Index Array")) -> ()
                n278 = global write "CRYProject Editor Global.vi" "Sequence Index for Calibration"(w425) -> ()
                n279 = global write "CRYProject Editor Global.vi" "Sequence Index for Hardware"(w425) -> ()
                n280 = case shown="False" w426 {
                  tunnel: w426 -> [_ w437]
                  frame False {
                    w430 = TRUE ("Visible")
                    w433 = FALSE ("Visible")
                    n281 = local read "Seq cont border Ref"() -> (w436:refnum<vi>)
                    n282 = local read "Seq Continue Ref"() -> (w435:refnum<vi>)
                    n283 = local read "Seq running Ref"() -> (w434:refnum<vi>)
                    n284 = property on="Continue" class="Bool (strict)"("Visible"=w430) -> ()  [unwired: 2 in, 2 out]
                    n285 = global write "CRYStatistics Global.vi" "RunStatisticsIndex Array"(u16[][] [] ("RunStatisticsIndex Array")) -> ()
                    n286 = Select(t=u8 0, s=w430, f=u8 2) -> (s? t:f=w429:u8)
                    n287 = property on="cont border" class="Bool (strict)"("Visible"=w430) -> ()  [unwired: 2 in, 2 out]
                    n288 = property class="Bool"(reference=w436, "Visible"=w430) -> ()  [unwired: 1 in, 2 out]
                    n289 = property class="Bool"(reference=w434, "Visible"=w433) -> ()  [unwired: 1 in, 2 out]
                    n290 = property on="running" class="Bool (strict)"("Visible"=w433) -> ()  [unwired: 2 in, 2 out]
                    n291 = property class="Bool"(reference=w435, "DisabledEnum"=w429) -> ()  [unwired: 1 in, 2 out]
                  }
                  frame True {
                    n292 = local read "Seq Continue Ref"() -> (w438:refnum<vi>)
                    n293 = local write "Continue"(w437) -> ()
                    n294 = property class="Bool"(reference=w438, "Value"=w437) -> ()  [unwired: 1 in, 2 out]
                  }
                }
                n295 = global write "CRYProject Editor Global.vi" "Step Setup VI No"(w427) -> ()
              }
              frame #2 {
                n296 = local read "Updateflg"() -> (w439:bool)
                n297 = case shown="False" w439 {
                  frame False {
                    n298 = global read "CRYCal Global.vi" "Calibrate"() -> (w440:bool)
                    n299 = case shown="False" w440 {
                      frame False {
                        n300 = call "CRYUpdate Steps Input Control.vi"() -> ()  [unwired: 12 in]
                        n301 = call "CRYUpdate Sequence Run.vi"("sOption"="AllUpdate") -> ()  [unwired: 11 in]
                      }
                      frame True {
                      }
                    }
                  }
                  frame True {
                  }
                }
              }
            }
          }
        }
      }
    }
    n302 = global read "CRYProject Run Control Global.vi" "RunState"() -> (w79:bool)
    n303 = global read "CRYProject Run Control Global.vi" "Aborted"() -> (w75:bool)
    n304 = global read "CRYMainGlobal.vi" "STOP"() -> (w77:bool)
    n305 = Not(x=w79) -> (.not. x?=w78:bool)
    n306 = Compound Arithmetic op=OR(w76, w75, w78, w77) -> (w73:bool)
  }
  n307 = flat-sequence {
    tunnel: w1 -> [_]
    frame #0 {
      n308 = global read "CRYCal Global.vi" "Calibrate"() -> (w446:bool)
      n309 = case shown="False" w446 {
        frame False {
          n310 = disable-structure shown="Disabled" {
            frame Disabled {
              n311 = global read "CRYData & result stacks global.vi" "Pause"() -> (w447:bool)
              n312 = case shown="False" w447 {
                frame False {
                  n313 = global read "CRYData & result stacks global.vi" "Redo"() -> (w448:bool)
                  n314 = case shown="False" w448 {
                    frame False {
                      n315 = global read "CRYData & result stacks global.vi" "Tested # No sum"() -> (w450:u16)
                      n316 = global read "CRYData & result stacks global.vi" "Tested #"() -> (w452:u16)
                      n317 = Increment(x=w452) -> (x+1=w451:u16)
                      n318 = Increment(x=w450) -> (x+1=w449:u16)
                      n319 = global write "CRYData & result stacks global.vi" "Tested #"(w451) -> ()
                      n320 = global write "CRYData & result stacks global.vi" "Tested # No sum"(w449) -> ()
                    }
                    frame True {
                    }
                  }
                }
                frame True {
                }
              }
            }
            frame Enabled {
            }
          }
        }
        frame True {
          n321 = global write "CRYProject Editor Global.vi" "Calibration TS Array"(T2 {"No.TS"=0, "TS File Path"=path "", "TS Name"="", "EditStepName"="", "Steps"=[], "New State"=FALSE, "Change State"=FALSE, "Flattened CurveLib Data"="", "Document Data"="", "EditStepNo"=0, "Operator Start File"="", "Sequence Type"="", "Sequence Language"=""} ("Calibration Cluster")) -> ()
        }
      }
      n322 = global read "CRYMain Sub Window Global.vi" "Main VI Ref"() -> (w442:refnum<vi>)
      n323 = call "CRYSet TooBar and StatusBar.vi"("Type"="EndSeq", "MainVI Ref In"=w442) -> ()  [unwired: 7 in, 3 out]
      n324 = control-ref of="This VI"() -> (w444:refnum<vi>)
      n325 = property class="VI"(reference=w444, "Front Panel.Open"=FALSE ("Front Panel Window:Open")) -> ()  [unwired: 1 in, 2 out]
    }
    frame #1 {
      w454 = FALSE ("Set Value")
      n326 = call "CRYInitialize Statistic Data.vi"() -> ()  [unwired: 12 in]
      n327 = call "CRYInit Data & result stacks global.vi"("Set Value"=TRUE, "No Project Exist?"=w454, "Pause Proc"=w454, "Init?"=w454) -> ()  [unwired: 8 in]
    }
    frame #2 {
      w456 = FALSE ("RunState")
      n328 = global read "CRYCal Global.vi" "Calibration Mic"() -> (w457:bool)
      n329 = global write "CRYData & result stacks global.vi" "Redo"(w456) -> ()
      n330 = global write "CRYProject Run Control Global.vi" "Cont Seq"(w456) -> ()
      n331 = global write "CRYProject Run Control Global.vi" "Cont State"(w456) -> ()
      n332 = global write "CRYProject Run Control Global.vi" "RunState"(w456) -> ()
      n333 = global write "CRYProject Run Control Global.vi" "Aborted"(w456) -> ()
      n334 = global write "CRYCal Global.vi" "Calibration Mic"(w456) -> ()
      n335 = global write "CRYProject Run Control Global.vi" "Run Stim steps only?"(w456) -> ()
      n336 = case shown="False" w457 {
        frame False {
          n337 = call "CRYInitialize Menu State.vi"("sAction"="Seq Stop", "Is Disable?"=FALSE) -> ()  [unwired: 10 in]
          n338 = call "CRYSet Enable Disable for Run.vi"("sOption"="Enable") -> ()  [unwired: 15 in]
          n339 = call "CRYAPI WSYSTEM.vi"("sAction"="PROJECT_STOP") -> ()  [unwired: 7 in, 4 out]
        }
        frame True {
        }
      }
    }
  }
